vi "Sim RC RL.vi"(11 "RC/RL Sim Param":refnum<vi>) -> (0 "Sampling Rate":dbl, 1 "Control Signal":dbl[](array[numeric]), 2 "Voltage Signal":dbl[](array[numeric]), 3 "Current Signal":dbl[](array[numeric]))   [LabVIEW 2014]
uses:
  <vilib>/measure/NI_MABase.lvlib
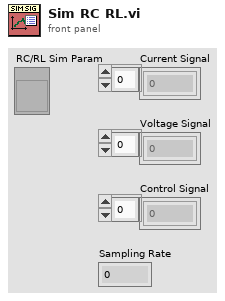
[diagram p1: front panel]
types:
  T1 = typedef "RCSim Controls.ctl" = cluster{"V":dbl, "C":dbl, "R":dbl, "L":dbl, "RC/RL":bool, "F":dbl, "DCycle":dbl}
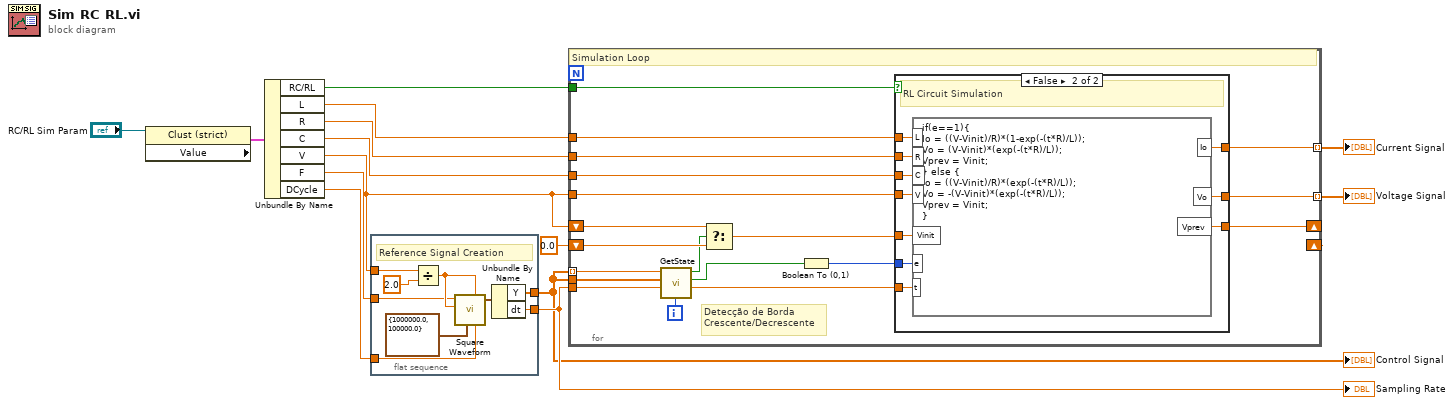
[diagram p0: block diagram]
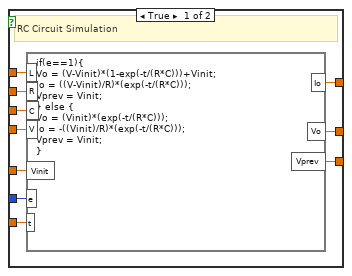
[diagram p2: hidden frame]
diagram:
  n1 = property class="Clust (strict)"(reference="RC/RL Sim Param") -> ("Value"=w9:T1)  [unwired: 1 in, 2 out]
  n2 = Unbundle By Name(w9) -> ("RC/RL"=w8:bool, "L"=w2:dbl, "R"=w3:dbl, "C"=w4:dbl, "V"=w5:dbl, "F"=w6:dbl, "DCycle"=w7:dbl)
  n3 = flat-sequence {
    tunnel: w5 -> [w19]
    tunnel: w6 -> [w18]
    tunnel: w7 -> [w17]
    tunnel: [w16] -> w11
    tunnel: [w15] -> w12
    frame #0 {
      # "Reference Signal Creation"
      n4 = Divide(x=w19, y=2.0) -> (x/y=w21:dbl)
      n5 = call <vilib>:"Square Waveform.vi"("duty cycle (%)"=w17, "offset"=w21, "sampling info"=cluster{"Fs":dbl, "#s":dbl} {"Fs"=1000000.0, "#s"=100000.0}, "amplitude"=w21, "frequency"=w18) -> ("signal out"=w20:waveform(dbl))  [unwired: 5 in, 1 out]
      n6 = Unbundle By Name(w20) -> ("Y"=w16:dbl[], "dt"=w15:dbl)
    }
  }
  n7 = for {
    tunnel: w3 -> [w42]
    tunnel: w4 -> [w41]
    tunnel: w5 -> [w37]
    tunnel: [w38] -> w14 mode=indexing
    tunnel: w11 -> [w39] mode=indexing
    tunnel: w11 -> [w40]
    shift-right: [w38] -> _
    shift-left: 0.0 ("y") -> [w33]
    shift-right: [w29] -> _
    shift-left: w5 -> [w32]
    tunnel: w12 -> [w35]
    tunnel: w2 -> [w28]
    tunnel: [w27] -> w13 mode=indexing
    tunnel: w8 -> [w24]
    i -> [w36]
    # "Detecção de Borda\nCrescente/Decrescente"
    # "Simulation Loop"
    n8 = call "GetState.vi"("Array Element"=w39, "Array"=w40, "dt"=w35, "Loop Iteration"=w36) -> ("Change State"=w31:bool, "Rising/Falling Edge"=w26:bool, "t"=w34:dbl)  [unwired: 3 in]
    n9 = Select(t=w32, s=w31, f=w33) -> (s? t:f=w30:dbl)
    n10 = Boolean To (0,1)(Boolean=w26) -> (0, 1=w25:i16)
    n11 = case shown="False" w24 {
      tunnel: w42 -> [w52 w62]
      tunnel: w41 -> [w51 w61]
      tunnel: [w50 w60] -> w38
      tunnel: w37 -> [w49 w59]
      tunnel: w34 -> [w48 w58]
      tunnel: w30 -> [w47 w57]
      tunnel: [w46 w56] -> w29
      tunnel: w28 -> [w45 w55]
      tunnel: [w44 w54] -> w27
      tunnel: w25 -> [w43 w53]
      frame True {
        # "RC Circuit Simulation"
        n12 = formula code="if(e==1){\nVo = (V-Vinit)*(1-exp(-t/(R*C)))+Vinit;\nIo = ((V-Vinit)/R)*(exp(-t/(R*C)));\nVprev = Vinit;\n} else {\nVo = (Vinit)*(exp(-t/(R*C)));\nIo = -((Vinit)/R)*(exp(-t/(R*C)));\nVprev = Vinit;\n}"("R"=w52, "C"=w51, "V"=w49, "t"=w48, "Vinit"=w47, "L"=w45, "e"=w43) -> ("Vo"=w50:dbl, "Vprev"=w46:dbl, "Io"=w44:dbl)
      }
      frame False {
        # "RL Circuit Simulation"
        n13 = formula code="if(e==1){\nIo = ((V-Vinit)/R)*(1-exp(-(t*R)/L));\nVo = (V-Vinit)*(exp(-(t*R)/L));\nVprev = Vinit;\n} else {\nIo = ((V-Vinit)/R)*(exp(-(t*R)/L));\nVo = -(V-Vinit)*(exp(-(t*R)/L));\nVprev = Vinit;\n}"("R"=w62, "C"=w61, "V"=w59, "t"=w58, "Vinit"=w57, "L"=w55, "e"=w53) -> ("Vo"=w60:dbl, "Vprev"=w56:dbl, "Io"=w54:dbl)
      }
    }
  }
  "Voltage Signal" <- w14
  "Current Signal" <- w13
  "Sampling Rate" <- w12
  "Control Signal" <- w11
